vi "Close Form.vi"(8 "error in (no error)":errorcluster, 10 "Form Name":T1, 11 "Form Server in":refnum<class "Form Server.lvclass">) -> (0 "error out":errorcluster, 3 "Form Server out":refnum<class "Form Server.lvclass">)   [LabVIEW 2020, in "Form Server.lvlib" / "Form Server.lvclass"]
uses:
  Form Server.lvclass
  Autoclose manager/Form ID.ctl
  Form Server.lvclass/Form Server.ctl
  Form Server Configuration/Form Server Configuration.lvclass/Form Server Configuration.ctl
  <vilib>/ActorFramework/Message Enqueuer/Message Enqueuer.lvclass/Message Enqueuer.ctl
  <vilib>/ActorFramework/Message Enqueuer/Enqueue.vi
  <vilib>/ActorFramework/Stop Msg/Stop Msg.lvclass
  C:/Program Files (x86)/National Instruments/LabVIEW 2020/vi.lib/ActorFramework/Message/Message.lvclass
  <vilib>/ActorFramework/Message Priority Queue/Priority Enqueue.vi
  Autoclose manager/Open Close Logic.lvclass
  Form Server Configuration/Form Server Configuration.lvclass
  Form Server Interfaces.lvlib
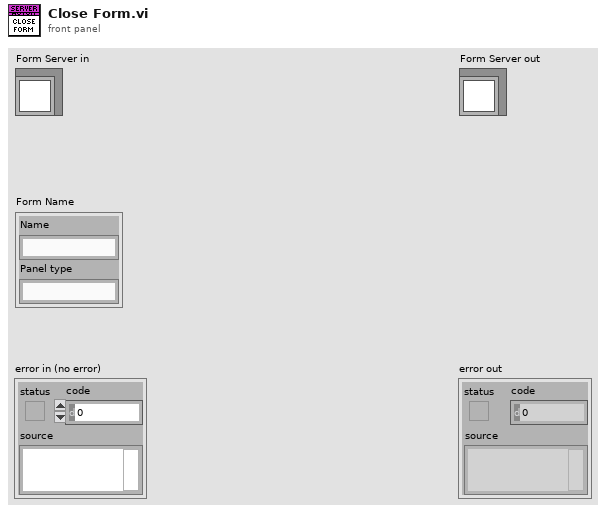
[diagram p1: front panel]
types:
  T1 = typedef "Form Server Interfaces.lvlib/Form ID.ctl" = cluster{"Name":string, "Panel type":string}
  T2 = map{T1, refnum<class "Message Enqueuer.lvclass">}
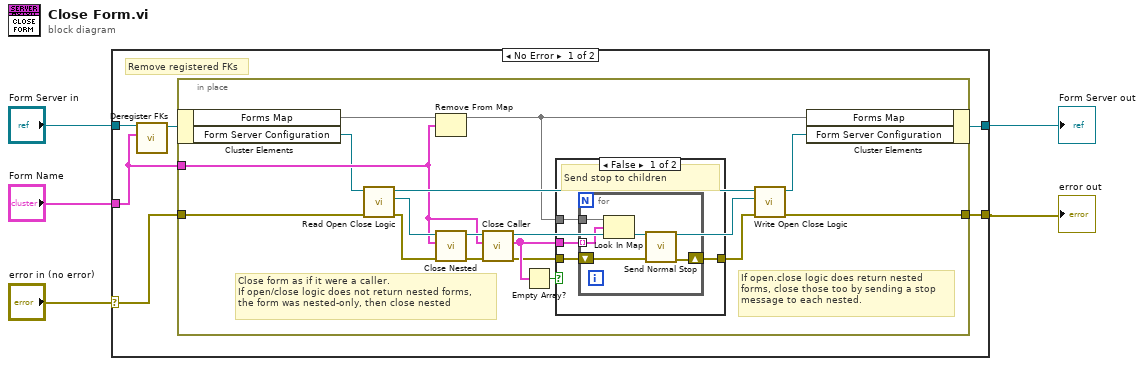
[diagram p0: block diagram]
diagram:
  n1 = case shown="No Error" "error in (no error)" {
    selector: "error in (no error)" -> [w11 w40]
    tunnel: [w10 w40] -> w1
    tunnel: [w6 w39] -> w3
    tunnel: "Form Server in" -> [w9 w39]
    tunnel: "Form Name" -> [w8 _]
    frame No Error {
      # "Remove registered FKs"
      n2 = call-dynamic "Deregister FKs.vi"("Form ID"=w8, "Form Server in"=w9) -> ("Form Server out"=w7:refnum<class "Form Server.lvclass">)  [unwired: 8 in, 1 out]
      n3 = in-place {
        in-place-border: w11 -> [w26]
        in-place-border: [w17] -> w10
        in-place-border: w8 -> [w16]
        # "If open.close logic does return nested forms, close those too by sending a stop message to each nested."
        # "Close form as if it were a caller.\nIf open/close logic does not return nested forms,\nthe form was nested-only, then close nested"
        n4 = in-place-cluster #1(w7) -> ("Forms Map"=w15:T2, "Form Server Configuration"=w14:refnum<class "Form Server Configuration.lvclass">)
        n5 = call "Read Open Close Logic.vi"("error in (no error)"=w26, "Form Server Configuration in"=w14) -> ("error out"=w18:errorcluster, "Form Server Interfaces.lvlib:Open Close Logic.lvclass"=w19:refnum<class "Open Close Logic.lvclass">, "Form Server Configuration out"=w24:refnum<class "Form Server Configuration.lvclass">)  [unwired: 7 in]
        n6 = Remove From Map(10:w16, 11:w15) -> (3:w12:T2)  [unwired: 2 out]
        n7 = call-dynamic "Close Nested.vi"("error in (no error)"=w18, "Nested"=w16, "Open Close Logic in"=w19) -> ("error out"=w20:errorcluster, "Open Close Logic out"=w21:refnum<class "Open Close Logic.lvclass">)  [unwired: 7 in]
        n8 = call-dynamic "Close Caller.vi"("error in (no error)"=w20, "Caller"=w16, "Open Close Logic in"=w21) -> ("error out"=w23:errorcluster, "Close Nested"=w27:T1[], "Open Close Logic out"=w22:refnum<class "Open Close Logic.lvclass">)  [unwired: 6 in]
        n9 = Empty Array?(array=w27) -> (empty?=w28:bool)
        n10 = case shown="False" w28 {
          tunnel: w27 -> [w32 _]
          tunnel: w12 -> [w31 _]
          tunnel: [w30 w38] -> w25
          tunnel: w23 -> [w29 w38]
          frame False {
            # "Send stop to children"
            n11 = for {
              tunnel: w32 -> [w36] mode=indexing
              tunnel: w31 -> [w37]
              shift-right: [w33] -> w30
              shift-left: w29 -> [w34]
              n12 = Look In Map(map=w37, key=w36) -> (value=w35:refnum<class "Message Enqueuer.lvclass">)  [unwired: 1 in, 1 out]
              n13 = call <vilib>:"Send Normal Stop.vi"("error in (no error)"=w34, "Message Enqueuer"=w35) -> ("error out"=w33:errorcluster)  [unwired: 9 in]
            }
          }
          frame True {
            # "No children forms"
          }
        }
        n14 = call "Write Open Close Logic.vi"("error in (no error)"=w25, "Form Server Interfaces.lvlib:Open Close Logic.lvclass"=w22, "Form Server Configuration in"=w24) -> ("error out"=w17:errorcluster, "Form Server Configuration out"=w13:refnum<class "Form Server Configuration.lvclass">)  [unwired: 7 in]
        n15 = in-place-cluster #1("Forms Map"=w12, "Form Server Configuration"=w13) -> (w6:refnum<class "Form Server.lvclass">)
      }
    }
    frame Error {
    }
  }
  "error out" <- w1
  "Form Server out" <- w3
